vi "PPL RT Driver VI_InlineHW.vi"(7 "Operation":T1, 11 "Device Reference in":T2 format="%.0x") -> (0 "Error Code":i32)   [LabVIEW 2020]
uses:
  <vilib>/NI VeriStand/Custom Device API/Custom Device Item Ref.ctl
  <vilib>/NI VeriStand/Custom Device API/Hardware Interface Driver VI Operation.ctl
  <vilib>/NI VeriStand/Custom Device API/Custom Device Channel Type.ctl
  <vilib>/NI VeriStand/Custom Device API/Data Reference.ctl
  <vilib>/NI VeriStand/Custom Device API/Data Access Type.ctl
  <vilib>/NI VeriStand/Custom Device API/Global Data Refs.vi
  <vilib>/NI VeriStand/Custom Device API/Custom Device API.lvlib
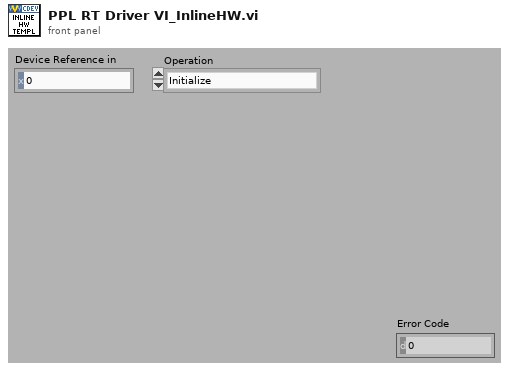
[diagram p1: front panel]
types:
  T1 = typedef "Custom Device API.lvlib/Hardware Interface Driver VI Operation.ctl" = enum16{"Initialize", "Start", "Read Data from HW", "Write Data to HW", "Close"}
  T2 = typedef "Custom Device API.lvlib/Custom Device Item Ref.ctl" = u64
  T3 = typedef "Custom Device API.lvlib/Data Reference.ctl" = i32
  T4 = cluster{"Input Values":dbl[], "Input Refs":T3[], "Output Values":dbl[], "Output Refs":T3[], "Device Error":errorcluster}
  T5 = typedef "Custom Device API.lvlib/Custom Device Channel Type.ctl" = enum16{"Input", "Output"}
  T6 = typedef "Custom Device API.lvlib/Data Access Type.ctl" = enum16{"Read", "Write"}
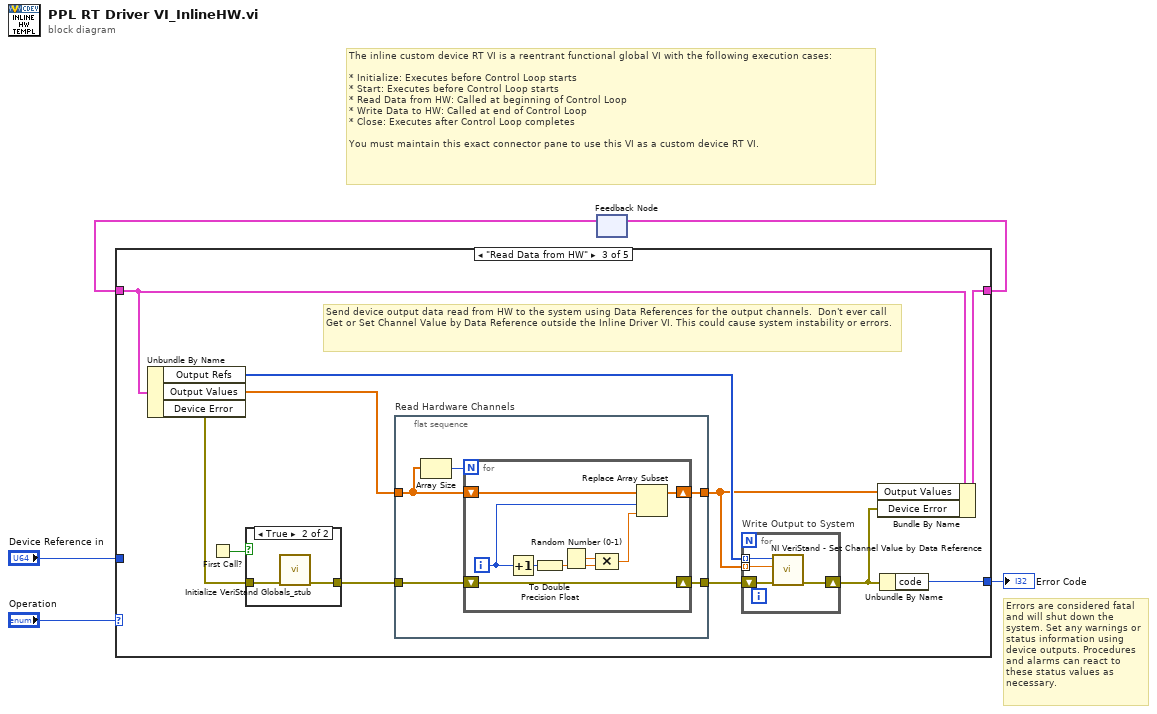
[diagram p0: block diagram]
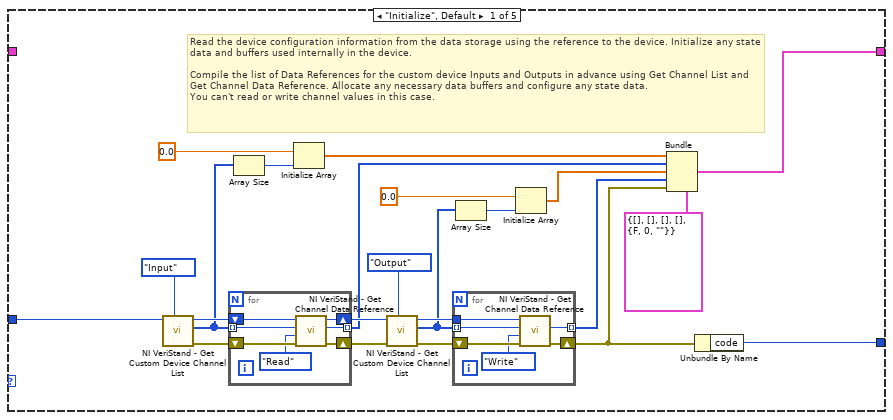
[diagram p2: hidden frame]
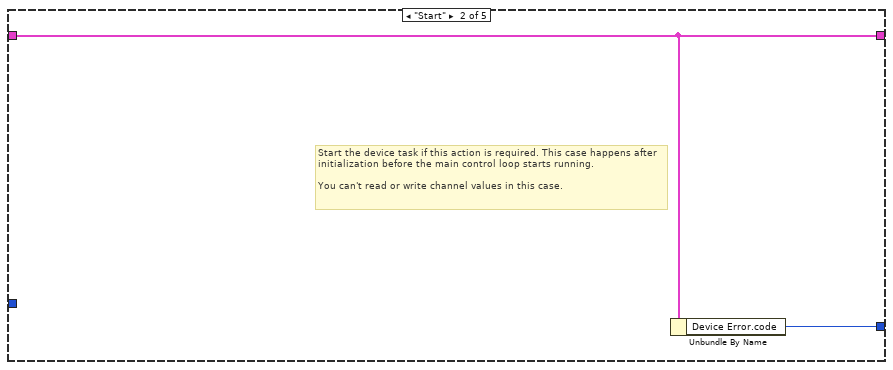
[diagram p3: hidden frame]
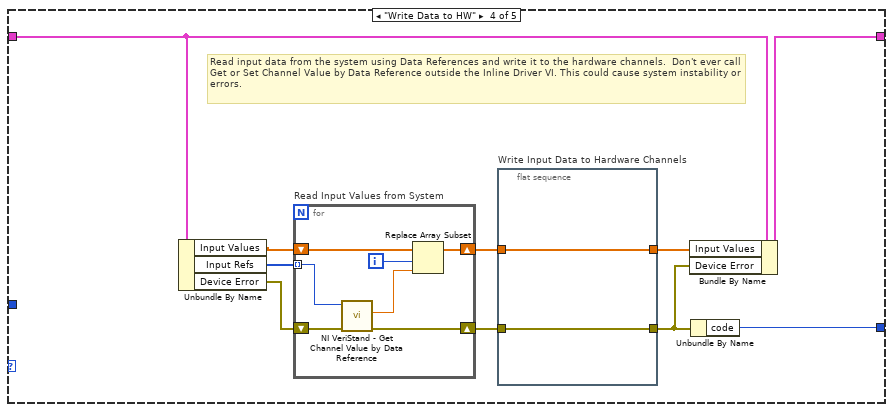
[diagram p5: hidden frame]
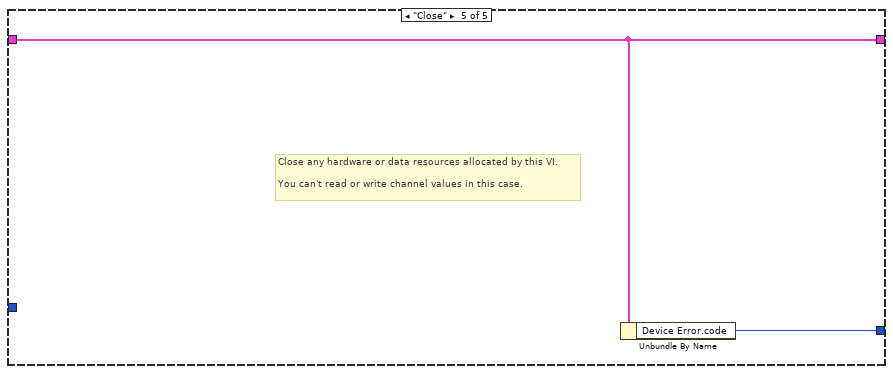
[diagram p6: hidden frame]
diagram:
  # "Errors are considered fatal and will shut down the system. Set any warnings or status information using device outputs. Procedures and alarms can react to these status values as necessary."
  # "The inline custom device RT VI is a reentrant functional global VI with the following execution cases:\n\n* Initialize: Executes before Control Loop starts\n* Start: Executes before Control Loop starts\n* Read Data from HW: Called at beginning of Control Loop\n* Write Data to HW: Called at end of Control Loop\n* Close: Executes after Control Loop completes\n\nYou must maintain this exact connector pane to use this VI as a custom device RT VI."
  n1 = feedback #1() -> (w3:T4)  [unwired: 1 out]
  n2 = case shown="\"Read Data from HW\"" "Operation" {
    tunnel: [w23 w42 w49 w83 w94] -> w4
    tunnel: w3 -> [_ w42 w50 w84 w94]
    tunnel: "Device Reference in" -> [w24 _ _ _ _]
    tunnel: [w22 w43 w53 w77 w95] -> w1
    frame "Initialize", Default {
      # "Read the device configuration information from the data storage using the reference to the device. Initialize any state data and buffers used internally in the device.\n\nCompile the list of Data References for the custom device Inputs and Outputs in advance using Get Channel List and Get Channel Data Reference. Allocate any necessary data buffers and configure any state data.\nYou can't read or write channel values in this case."
      n3 = call <vilib>:"NI VeriStand - Get Custom Device Channel List.vi"("Channel Type"=Custom_Device_Channel_Type."Input", "Device Ref in"=w24) -> ("error out"=w20:errorcluster, "Specified Channel Ref List"=w19:T2[], "Device Ref out"=w21:T2)  [unwired: 1 in, 6 out]
      n4 = for {
        shift-right: [w36] -> w15
        shift-left: w21 -> [w40]
        tunnel: w19 -> [w39] mode=indexing
        shift-right: [w37] -> w14
        shift-left: w20 -> [w41]
        tunnel: [w35] -> w13 mode=indexing
        n5 = call <vilib>:"NI VeriStand - Get Channel Data Reference.vi"("error in (no error)"=w41, "Access"=Data_Access_Type."Read", "Channel Ref in"=w39, "Device Ref in"=w40) -> ("error out"=w37:errorcluster, "Channel Data Reference"=w35:T3, "Device Ref out"=w36:T2)  [unwired: 5 out]
      }
      n6 = Array Size(array=w19) -> (size(s)=w27:i32)
      n7 = Initialize Array(0.0 ("element"), w27) -> (w28:dbl[])
      n8 = call <vilib>:"NI VeriStand - Get Custom Device Channel List.vi"("Channel Type"=Custom_Device_Channel_Type."Output", "error in (no error)"=w14, "Device Ref in"=w15) -> ("error out"=w18:errorcluster, "Specified Channel Ref List"=w10:T2[], "Device Ref out"=w17:T2)  [unwired: 6 out]
      n9 = for {
        tunnel: w10 -> [w32] mode=indexing
        shift-right: [w30] -> w6
        shift-left: w18 -> [w34]
        tunnel: [w29] -> w8 mode=indexing
        tunnel: w17 -> [w33]
        n10 = call <vilib>:"NI VeriStand - Get Channel Data Reference.vi"("error in (no error)"=w34, "Access"=Data_Access_Type."Write", "Channel Ref in"=w32, "Device Ref in"=w33) -> ("error out"=w30:errorcluster, "Channel Data Reference"=w29:T3)  [unwired: 6 out]
      }
      n11 = Array Size(array=w10) -> (size(s)=w11:i32)
      n12 = Initialize Array(0.0 ("element"), w11) -> (w9:dbl[])
      n13 = Bundle(cluster=T4 {"Input Values"=[], "Input Refs"=[], "Output Values"=[], "Output Refs"=[], "Device Error"={"status"=FALSE, "code"=0, "source"=""}}, "Input Values"=w28, "Input Refs"=w13, "Output Values"=w9, "Output Refs"=w8, "Device Error"=w6) -> (w23:T4)
      n14 = Unbundle By Name(w6) -> ("code"=w22:i32)
    }
    frame "Start" {
      # "Start the device task if this action is required. This case happens after initialization before the main control loop starts running.\n\nYou can't read or write channel values in this case."
      n15 = Unbundle By Name(w42) -> ("Device Error.code"=w43:i32)
    }
    frame "Read Data from HW" {
      # "Send device output data read from HW to the system using Data References for the output channels.  Don't ever call Get or Set Channel Value by Data Reference outside the Inline Driver VI. This could cause system instability or errors."
      n16 = Unbundle By Name(w50) -> ("Output Refs"=w52:T3[], "Output Values"=w51:dbl[], "Device Error"=w44:errorcluster)
      n17 = First Call?() -> (First Call?: T/F=w46:bool)
      n18 = case shown="True" w46 {
        tunnel: [w55 w56] -> w45
        tunnel: w44 -> [w55 w57]
        frame False {
        }
        frame True {
          n19 = call "Initialize VeriStand Globals_stub.vi"("error in (no error)"=w57) -> ("error out"=w56:errorcluster)  [unwired: 10 in]
        }
      }
      n20 = flat-sequence "Read Hardware Channels" {
        tunnel: w45 -> [w66]
        tunnel: [w65] -> w54
        tunnel: [w62] -> w48
        tunnel: w51 -> [w63]
        frame #0 {
          n21 = Array Size(array=w63) -> (size(s)=w64:i32)
          n22 = for {
            N: w64 -> [_]
            shift-right: [w71] -> w65
            shift-left: w66 -> [w71]
            shift-right: [w68] -> w62
            shift-left: w63 -> [w70]
            i -> [w67]
            n23 = Increment(x=w67) -> (x+1=w73:i32)
            n24 = To Double Precision Float(number=w73) -> (double precision float=w72:dbl)
            n25 = Random Number (0-1)() -> (number: 0 to 1=w74:dbl)
            n26 = Compound Arithmetic op=MULTIPLY(w74, w72) -> (w69:dbl)
            n27 = Replace Array Subset(array=w70, new element=w69, index=w67) -> (w68:dbl[])
          }
        }
      }
      n28 = for "Write Output to System" {
        shift-right: [w60] -> w47
        shift-left: w54 -> [w61]
        tunnel: w48 -> [w59] mode=indexing
        tunnel: w52 -> [w58] mode=indexing
        n29 = call <vilib>:"NI VeriStand - Set Channel Value by Data Reference.vi"("error in (no error)"=w61, "Value"=w59, "Data Reference in"=w58) -> ("error out"=w60:errorcluster)  [unwired: 8 out]
      }
      n30 = Bundle By Name(cluster=w50, "Output Values"=w48, "Device Error"=w47) -> (w49:T4)
      n31 = Unbundle By Name(w47) -> ("code"=w53:i32)
    }
    frame "Write Data to HW" {
      # "Read input data from the system using Data References and write it to the hardware channels.  Don't ever call Get or Set Channel Value by Data Reference outside the Inline Driver VI. This could cause system instability or errors."
      n32 = Unbundle By Name(w84) -> ("Input Values"=w81:dbl[], "Input Refs"=w82:T3[], "Device Error"=w76:errorcluster)
      n33 = for "Read Input Values from System" {
        shift-right: [w87] -> w78
        shift-left: w76 -> [w93]
        tunnel: w82 -> [w92] mode=indexing
        shift-right: [w90] -> w80
        shift-left: w81 -> [w91]
        i -> [w89]
        n34 = call <vilib>:"NI VeriStand - Get Channel Value by Data Reference.vi"("error in (no error)"=w93, "Data Reference in"=w92) -> ("error out"=w87:errorcluster, "Value"=w88:dbl)  [unwired: 8 out]
        n35 = Replace Array Subset(array=w91, new element=w88, index=w89) -> (w90:dbl[])
      }
      n36 = flat-sequence "Write Input Data to Hardware Channels" {
        tunnel: w80 -> [w86]
        tunnel: [w86] -> w79
        tunnel: [w85] -> w75
        tunnel: w78 -> [w85]
        frame #0 {
        }
      }
      n37 = Bundle By Name(cluster=w84, "Input Values"=w79, "Device Error"=w75) -> (w83:T4)
      n38 = Unbundle By Name(w75) -> ("code"=w77:i32)
    }
    frame "Close" {
      # "Close any hardware or data resources allocated by this VI.\n\nYou can't read or write channel values in this case."
      n39 = Unbundle By Name(w94) -> ("Device Error.code"=w95:i32)
    }
  }
  "Error Code" <- w1
  n40 = feedback-in #1(w4) -> ()
